vi "Get Server Address.vi"(11 "OOP Server in":refnum<class "Query Server.lvclass">) -> (2 "Server Address":string, 3 "OOP Server out":refnum<class "Query Server.lvclass">)   [LabVIEW 2016, in "Query Server.lvlib" / "Query Server.lvclass"]
uses:
  Query Server.lvclass
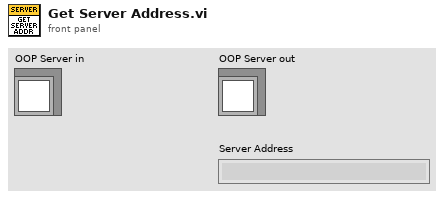
[diagram p1: front panel]
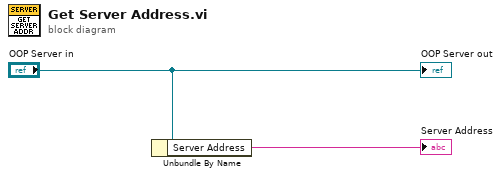
[diagram p0: block diagram]
diagram:
  n1 = Unbundle By Name("OOP Server in") -> ("Server Address"=→"Server Address":string)
  "OOP Server out" <- "OOP Server in"
